vi "Main.vi"(11 "Module Admin":refnum<class "Delacor_lib_QMH_Module Admin.lvclass">) -> ()   [LabVIEW 2019, in "Aquisition.lvlib"]
doc: "This template is based off of the Queued Message Handler design pattern and the Queued Message Handler project template that ships with LabVIEW.\n\nThe main difference is that the queue is private to this module and communication between modules is performed via Broadcast and Request events.\n\nRequest events are wrapped in public API methods and are handled in the Event Handling Loop (EHL) of this VI. Any module can register for Broadcast events sent by this module. The EHL generates messages based on user interface actions.\n\nThe Message Handling Loop (MHL) processes messages generated by the EHL, or by other messages. The messages are string values, so new messages can be added easily to the Message Cases case structure in the MHL. Each message cluster can also provide an optional value for Message Data, which is a variant that can be converted to whatever message-specific data is required.\n_____\nBased on Delacor QMH Project Template 5.0.0.82."
uses:
  Aquisition.lvlib
  <vilib>/Delacor/Delacor QMH/Libraries/Module Admin_class/Delacor_lib_QMH_Module Admin.lvclass
  Module Data--cluster.ctl
  <vilib>/Delacor/Delacor QMH/Libraries/Message Queue_class/Delacor_lib_QMH_Message Queue.lvclass/Delacor_lib_QMH_Message Queue.ctl
  Stop Argument--cluster.ctl
  <vilib>/Delacor/Delacor QMH/Libraries/Module Admin_class/Delacor_lib_QMH_Module Admin.lvclass/Delacor_lib_QMH_Module Admin.ctl
  <vilib>/Utility/miscctls.llb/LVPointTypeDef.ctl
  <vilib>/Delacor/Delacor QMH/Libraries/Message Queue_class/Delacor_lib_QMH_Enqueue Message (Single).vi
  <vilib>/Delacor/Delacor QMH/Libraries/Module Admin_class/Delacor_lib_QMH_Get External Launch.vi
  <vilib>/Utility/error.llb/Error Cluster From Error Code.vi
  <vilib>/ErrorRing/Error Ring.xnode
  <vilib>/Delacor/Delacor QMH/Libraries/Message Queue_class/Delacor_lib_QMH_Message Queue.lvclass
panel:
  in  "Simulate MHL Error":bool
  in  "Simulate EHL Error":bool
  out "error out":errorcluster
  out "Status":string
  # "Other QMH Modules communicate with this Module via its Public API (wrappers for its Request Events).\n\nThis Module communicates with other Modules via its Broadcast Events.\nAny module that wants to get these messages, just registers for this module's Broadcast events."
  # "This template is for the Delacor Modified Queued Message Handler design pattern.\n\nSee the block diagram for more information on how to use this template."
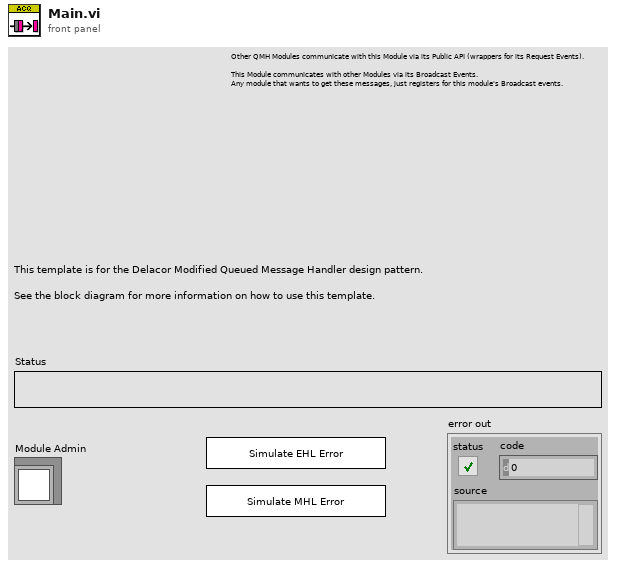
[diagram p1: front panel]
types:
  T1 = typedef "Aquisition.lvlib/Request Events--cluster.ctl" = cluster{"Stop Module":refnum<user-event>, "Show Panel":refnum<user-event>, "Hide Panel":refnum<user-event>, "Get Module Execution Status":refnum<user-event>, "Show Diagram":refnum<user-event>}
  T2 = typedef "Aquisition.lvlib/Module Data--cluster.ctl" = cluster{"Status":string}
  T3 = enum32{"invalid lock state", "Not Locked", "Locked (No Password)", "Password-protected"}
  T4 = typedef "Aquisition.lvlib/Stop Argument--cluster.ctl" = cluster{"Origin":string, "Exit via Stop Module Req?":bool, "Wait for Module to stop?":bool}
  T5 = typedef "LVPointTypeDef.ctl" = cluster{"Horizontal":i16, "Vertical":i16}
  T6 = enum32{"Invalid", "Standard", "Closed", "Hidden", "Minimized", "Maximized"}
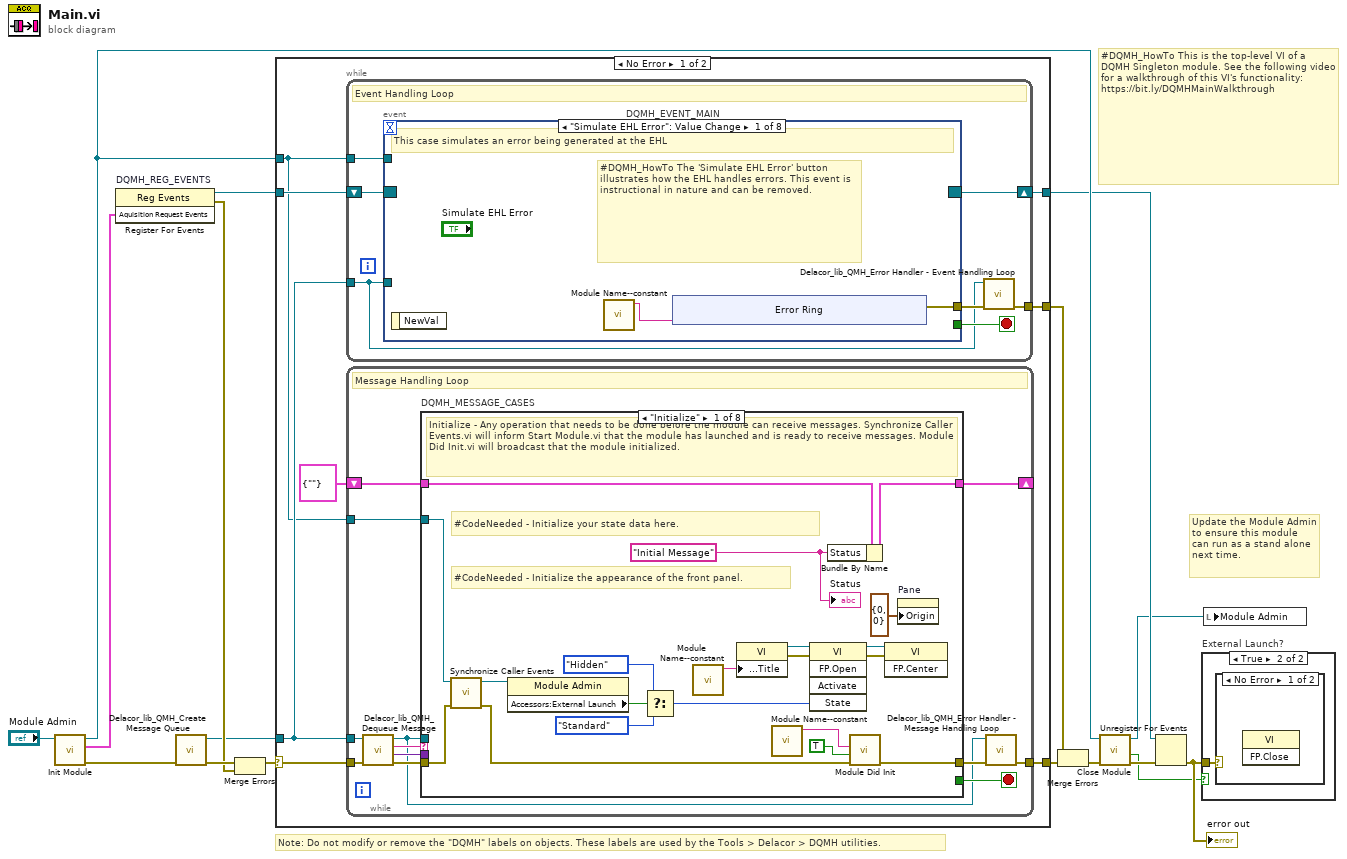
[diagram p0: block diagram]
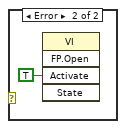
[diagram p3: hidden frame]
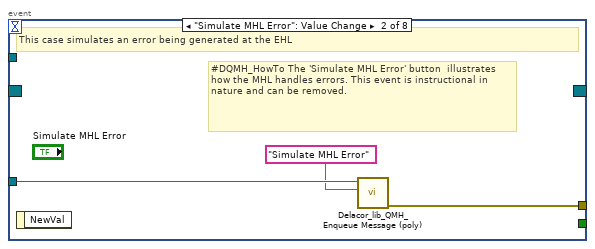
[diagram p4: hidden frame]
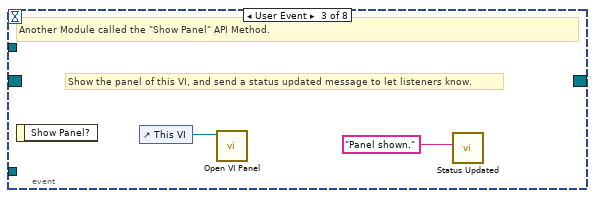
[diagram p5: hidden frame]
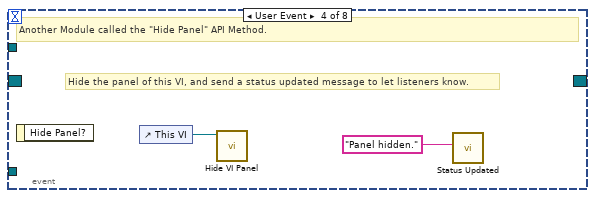
[diagram p6: hidden frame]
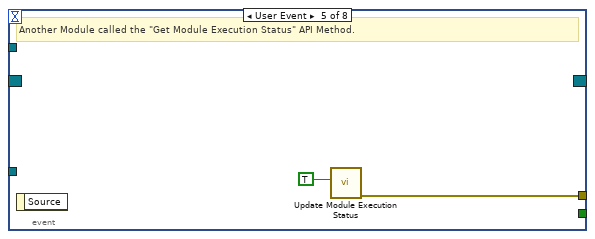
[diagram p7: hidden frame]
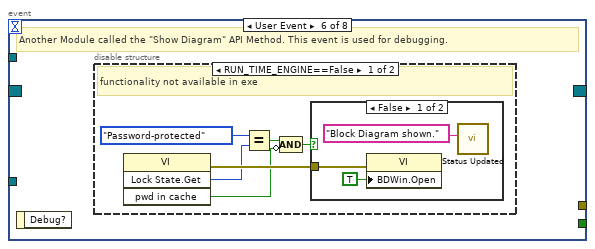
[diagram p8: hidden frame]
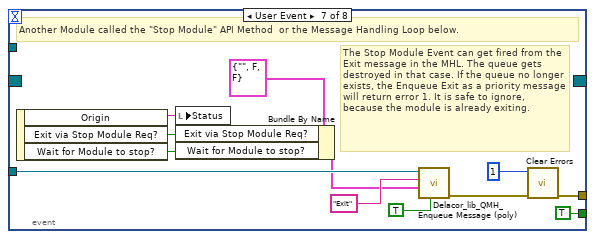
[diagram p11: hidden frame]
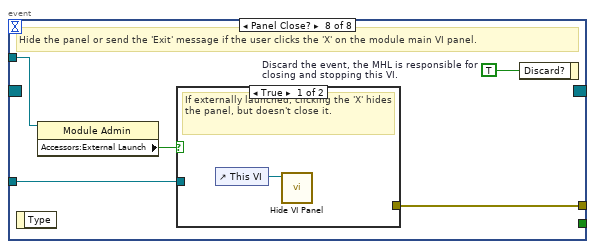
[diagram p12: hidden frame]
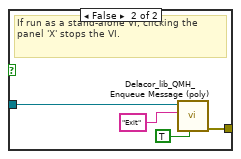
[diagram p13: hidden frame]
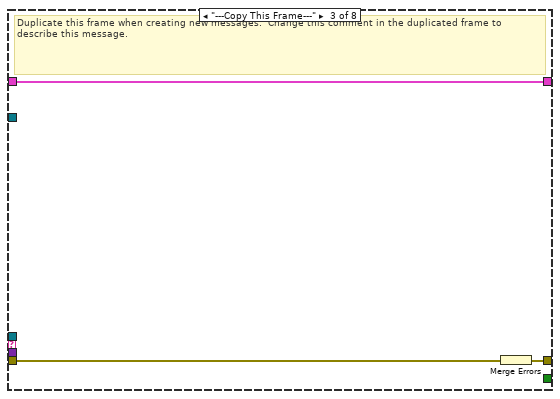
[diagram p15: hidden frame]
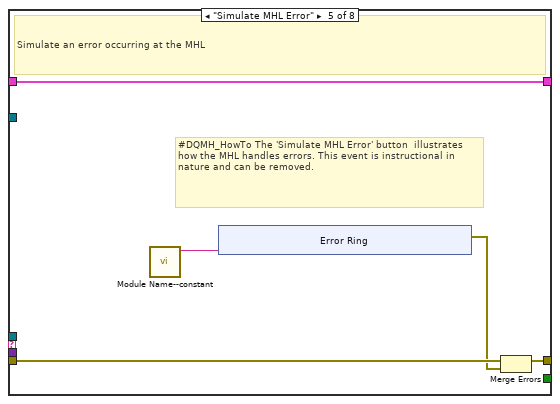
[diagram p17: hidden frame]
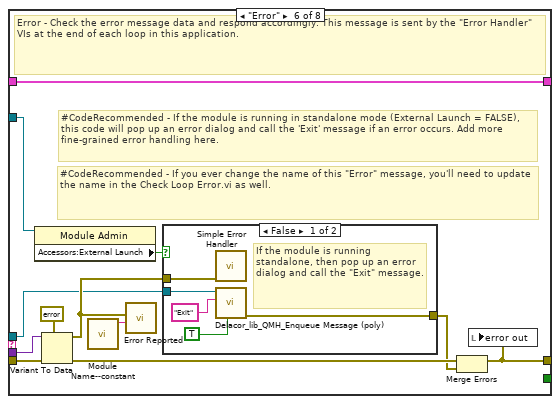
[diagram p18: hidden frame]
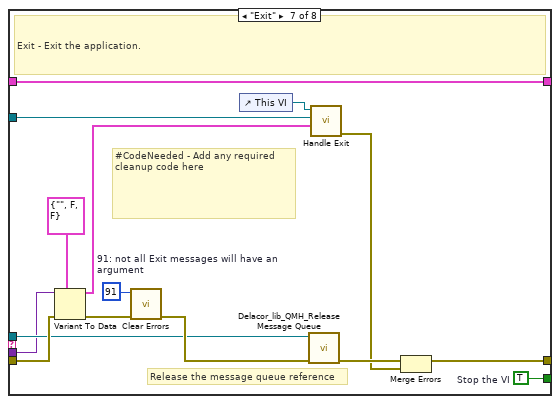
[diagram p20: hidden frame]
diagram:
  # "#DQMH_HowTo This is the top-level VI of a DQMH Singleton module. See the following video for a walkthrough of this VI's functionality: https://bit.ly/DQMHMainWalkthrough"
  # "Note: Do not modify or remove the \"DQMH\" labels on objects. These labels are used by the Tools > Delacor > DQMH utilities."
  # "Update the Module Admin to ensure this module can run as a stand alone next time."
  n1 = call "Init Module.vi"("Singleton Module Admin in"="Module Admin") -> ("error out"=w16:errorcluster, "Aquisition Request Events"=w5:T1, "Singleton Module Admin out"=w8:refnum<class "Delacor_lib_QMH_Module Admin.lvclass">)  [unwired: 8 in]
  n2 = register-events "DQMH_REG_EVENTS"(w5) -> (reference out=w6:refnum<event-registration>, error out=w9:errorcluster)  [unwired: 2 in]
  n3 = call <vilib>:"Delacor_lib_QMH_Create Message Queue.vi"("error in (no error)"=w16) -> ("error out"=w11:errorcluster, "Message Queue"=w4:refnum<class "Delacor_lib_QMH_Message Queue.lvclass">)  [unwired: 9 in]
  n4 = Merge Errors(w11, w9) -> (w10:errorcluster)
  n5 = case shown="No Error" w10 {
    selector: w10 -> [w23 w181]
    tunnel: [w25 w180] -> w17
    tunnel: [w22 w186] -> w7
    tunnel: w6 -> [w20 w186]
    tunnel: w4 -> [w19 w179]
    tunnel: [w24 _] -> w14
    tunnel: w8 -> [w18 w182]
    frame No Error {
      n6 = while {
        tunnel: w19 -> [w26]
        shift-right: [w29] -> w22
        shift-left: w20 -> [w30]
        tunnel: [w31] -> w24
        tunnel: w18 -> [w27]
        stop <- w28 stop-if-true
        # "Event Handling Loop"
        n7 = event "DQMH_EVENT_MAIN" shown="[0] \"Simulate EHL Error\": Value Change" {
          selector: w30 -> [_ _ _ _ _ _ _ _]
          dyn-events: [_ _ _ _ _ _ _ _] -> w29
          timeout: _ -> [_ _ _ _ _ _ _ _]
          tunnel: [_ _ _ _ _ _ TRUE ("Discard?") _] -> w28
          tunnel: w26 -> [_ w43 _ _ _ _ w67 w74]
          tunnel: [w34 w44 _ _ w50 _ w70 w76] -> w32
          tunnel: w27 -> [_ _ _ _ _ _ _ w73]
          event "Simulate EHL Error": Value Change {
            # "#DQMH_HowTo The 'Simulate EHL Error' button  illustrates how the EHL handles errors. This event is instructional in nature and can be removed."
            # "This case simulates an error being generated at the EHL"
            n8 = event-data() -> ()  [unwired: 1 in, 1 out]
            n9 = call "Module Name--constant.vi"() -> ("Module Name"=w33:string)  [unwired: 11 in]
            n10 = xnode "Error Ring"("parameter 0"=w33) -> ("error out"=w34:errorcluster)
          }
          event "Simulate MHL Error": Value Change {
            # "#DQMH_HowTo The 'Simulate MHL Error' button  illustrates how the MHL handles errors. This event is instructional in nature and can be removed."
            # "This case simulates an error being generated at the EHL"
            n11 = event-data() -> ()  [unwired: 1 in, 1 out]
            n12 = call-poly <vilib>:"Delacor_lib_QMH_Enqueue Message (poly).vi"("Message"="Simulate MHL Error", "Message Queue in"=w43) -> ("error out"=w44:errorcluster)  [unwired: 8 in, 1 out]
          }
          event User Event {
            # "Show the panel of this VI, and send a status updated message to let listeners know."
            # "Another Module called the \"Show Panel\" API Method."
            n13 = event-data() -> ()  [unwired: 1 in, 1 out]
            n14 = control-ref of="This VI"() -> (w46:refnum<vi>)
            n15 = call "Open VI Panel.vi"("VI"=w46) -> ()  [unwired: 10 in, 1 out]
            n16 = call "Status Updated.vi"("Status"="Panel shown." ("format string")) -> ()  [unwired: 10 in, 1 out]
          }
          event User Event {
            # "Hide the panel of this VI, and send a status updated message to let listeners know."
            # "Another Module called the \"Hide Panel\" API Method."
            n17 = event-data() -> ()  [unwired: 1 in, 1 out]
            n18 = control-ref of="This VI"() -> (w48:refnum<vi>)
            n19 = call "Hide VI Panel.vi"("VI"=w48) -> ()  [unwired: 10 in, 1 out]
            n20 = call "Status Updated.vi"("Status"="Panel hidden." ("format string")) -> ()  [unwired: 10 in, 1 out]
          }
          event User Event {
            # "Another Module called the \"Get Module Execution Status\" API Method."
            n21 = event-data() -> ()  [unwired: 1 in, 1 out]
            n22 = call "Update Module Execution Status.vi"("Running?"=TRUE) -> ("error out"=w50:errorcluster)  [unwired: 10 in]
          }
          event User Event {
            # "Another Module called the \"Show Diagram\" API Method. This event is used for debugging."
            n23 = event-data() -> ()  [unwired: 1 in, 1 out]
            n24 = disable-structure shown="RUN_TIME_ENGINE==False" {
              frame condition #0 (active) {
                # "functionality not available in exe"
                n25 = invoke class="VI" method="Lock State.Get"() -> (error out=w56:errorcluster, "Get Lock State"=w55:T3, "pwd in cache"=w52:bool)  [unwired: 4 in, 1 out]
                n26 = Equal?(x=T3."Password-protected", y=w55) -> (x = y?=w53:bool)
                n27 = Compound Arithmetic op=AND(w53, invert w52) -> (w51:bool)
                n28 = case shown="False" w51 {
                  tunnel: w56 -> [w59 _]
                  frame False {
                    n29 = property class="VI"(error in=w59, "BDWin.Open"=TRUE ("Block Diagram Window:Open")) -> ()  [unwired: 1 in, 2 out]
                    n30 = call "Status Updated.vi"("Status"="Block Diagram shown." ("format string")) -> ()  [unwired: 10 in, 1 out]
                  }
                  frame True {
                    # "Password-protected VI, and the password is not in the cache. Do not show the diagram."
                  }
                }
              }
              frame condition #1 {
              }
            }
          }
          event User Event {
            # "The Stop Module Event can get fired from the Exit message in the MHL. The queue gets destroyed in that case. If the queue no longer exists, the Enqueue Exit as a priority message will return error 1. It is safe to ignore, because the module is already exiting."
            # "Another Module called the \"Stop Module\" API Method  or the Message Handling Loop below."
            n31 = event-data() -> ("Origin"=w66:string, "Exit via Stop Module Req?"=w62:bool, "Wait for Module to stop?"=w61:bool)  [unwired: 1 in]
            n32 = local write "Status"(w66) -> ()
            n33 = Bundle By Name(cluster=T4 {"Origin"="", "Exit via Stop Module Req?"=FALSE, "Wait for Module to stop?"=FALSE} ("Stop Argument"), "Exit via Stop Module Req?"=w62, "Wait for Module to stop?"=w61) -> (w60:T4)
            n34 = call-poly <vilib>:"Delacor_lib_QMH_Enqueue Message (poly).vi"("Priority Message? (F)"=TRUE, "Message Data"=w60, "Message"="Exit", "Message Queue in"=w67) -> ("error out"=w71:errorcluster)  [unwired: 6 in, 1 out]
            n35 = call <vilib>:"Clear Errors.vi"("error in (no error)"=w71, "specific error code to clear (0: all)"=1) -> ("error out"=w70:errorcluster)  [unwired: 4 in, 1 out]
          }
          event Panel Close? {
            w75 = TRUE  # Discard the event, the MHL is responsible for closing and stopping this VI.
            # "Hide the panel or send the 'Exit' message if the user clicks the 'X' on the module main VI panel."
            n36 = event-data() -> ()  [unwired: 1 in, 1 out]
            n37 = property class="Module Admin"(reference=w73) -> ("Accessors:External Launch"=w72:bool)  [unwired: 1 in, 2 out]
            n38 = case shown="True" w72 {
              tunnel: w74 -> [_ w80]
              tunnel: [_ w81] -> w76
              frame True {
                # "If externally launched, clicking the 'X' hides the panel, but doesn't close it."
                n39 = control-ref of="This VI"() -> (w77:refnum<vi>)
                n40 = call "Hide VI Panel.vi"("VI"=w77) -> ()  [unwired: 10 in, 1 out]
              }
              frame False {
                # "If run as a stand-alone VI, clicking the panel 'X' stops the VI."
                n41 = call-poly <vilib>:"Delacor_lib_QMH_Enqueue Message (poly).vi"("Priority Message? (F)"=TRUE, "Message"="Exit", "Message Queue in"=w80) -> ("error out"=w81:errorcluster)  [unwired: 7 in, 1 out]
              }
            }
            n42 = event-data("Discard?"=w75) -> ()  [unwired: 1 in, 1 out]
          }
        }
        n43 = call-dynamic "Delacor_lib_QMH_Error Handler - Event Handling Loop.vi"("error in (no error)"=w32, "Message Queue in"=w26) -> ("dup error in"=w31:errorcluster)  [unwired: 8 in, 1 out]
      }
      n44 = while {
        tunnel: w19 -> [w84]
        shift-right: [w88] -> _
        shift-left: T2 {"Status"=""} ("Data Cluster") -> [w89]
        tunnel: w23 -> [w92]
        tunnel: [w90] -> w25
        tunnel: w18 -> [w82]
        stop <- w87 stop-if-true
        # "Message Handling Loop"
        n45 = call-dynamic "Delacor_lib_QMH_Dequeue Message.vi"("error in (no error)"=w92, "Message Queue in"=w84) -> ("error out"=w91:errorcluster, "Message Data"=w85:variant, "Message"=w86:string, "Message Queue out"=w83:refnum<class "Delacor_lib_QMH_Message Queue.lvclass">)  [unwired: 6 in]
        n46 = case "DQMH_MESSAGE_CASES" shown="\"Initialize\"" w86 {
          selector: w86 -> [_ _ _ _ _ _ _ w166]
          tunnel: w83 -> [_ _ _ _ _ w136 w158 _]
          tunnel: w91 -> [w111 w115 w118 w120 w125 w143 w164 w168]
          tunnel: [w109 w115 w117 w120 w124 w139 w161 w169] -> w93
          tunnel: w89 -> [w100 w114 w116 w119 w122 w138 w157 w167]
          tunnel: [w99 w114 w116 w119 w122 w138 w157 w167] -> w88
          tunnel: [_ _ _ _ _ _ w156 _] -> w87
          tunnel: w85 -> [_ _ _ _ _ w137 w155 _]
          tunnel: w82 -> [w101 _ _ _ _ w135 w150 _]
          frame "Initialize" {
            w94 = "Initial Message" ("Initial Message")
            # "#CodeNeeded - Initialize the appearance of the front panel."
            # "#CodeNeeded - Initialize your state data here."
            # "Initialize - Any operation that needs to be done before the module can receive messages. Synchronize Caller Events.vi will inform Start Module.vi that the module has launched and is ready to receive messages. Module Did Init.vi will broadcast that the module initialized."
            n47 = call "Synchronize Caller Events.vi"("error in (no error)"=w111, "Singleton Module Admin in"=w101) -> ("error out"=w110:errorcluster, "Singleton Module Admin out"=w96:refnum<class "Delacor_lib_QMH_Module Admin.lvclass">)  [unwired: 8 in]
            n48 = property class="Module Admin"(reference=w96) -> ("Accessors:External Launch"=w105:bool)  [unwired: 1 in, 2 out]
            n49 = Select(t=T6."Hidden" ("State"), s=w105, f=T6."Standard" ("State")) -> (s? t:f=w102:T6)
            n50 = call "Module Name--constant.vi"() -> ("Module Name"=w108:string)  [unwired: 11 in]
            n51 = property class="VI"("Front Panel.Title"=w108) -> (reference out=w107:refnum<vi>, error out=w113:errorcluster)  [unwired: 2 in]
            n52 = call "Module Name--constant.vi"() -> ("Module Name"=w97:string)  [unwired: 11 in]
            n53 = invoke class="VI" method="FP.Open"(reference=w107, error in=w113, "State"=w102) -> (reference out=w106:refnum<vi>, error out=w112:errorcluster)  [unwired: 2 in, 3 out]
            n54 = Bundle By Name(cluster=w100, "Status"=w94) -> (w99:T2)
            n55 = call "Module Did Init.vi"("error in (no error)"=w110, "Initialized?"=TRUE, "Origin"=w97) -> ("error out"=w109:errorcluster)  [unwired: 8 in]
            n56 = invoke class="VI" method="FP.Center"(reference=w106, error in=w112) -> ()  [unwired: 1 in, 3 out]
            n57 = property on="Pane" class="Pane"("Origin"=T5 {"Horizontal"=0, "Vertical"=0}) -> ()  [unwired: 2 in, 2 out]
            "Status" <- w94
          }
          frame "--- Module Specific ---" {
            # "Separator -- The following cases handle messages specific to this Module."
          }
          frame "---Copy This Frame---" {
            # "Duplicate this frame when creating new messages.  Change this comment in the duplicated frame to describe this message."
            n58 = Merge Errors(w118) -> (w117:errorcluster)
          }
          frame "--- Exit and Error Handling---" {
            # "Separator - The following cases handle errors and exit messages."
          }
          frame "Simulate MHL Error" {
            # "#DQMH_HowTo The 'Simulate MHL Error' button  illustrates how the MHL handles errors. This event is instructional in nature and can be removed."
            # "Simulate an error occurring at the MHL"
            n59 = call "Module Name--constant.vi"() -> ("Module Name"=w121:string)  [unwired: 11 in]
            n60 = xnode "Error Ring"("parameter 0"=w121) -> ("error out"=w123:errorcluster)
            n61 = Merge Errors(w125, w123) -> (w124:errorcluster)
          }
          frame "Error" {
            # "#CodeRecommended - If you ever change the name of this \"Error\" message, you'll need to update the name in the Check Loop Error.vi as well."
            # "#CodeRecommended - If the module is running in standalone mode (External Launch = FALSE), this code will pop up an error dialog and call the 'Exit' message if an error occurs. Add more fine-grained error handling here."
            # "Error - Check the error message data and respond accordingly. This message is sent by the \"Error Handler\" VIs at the end of each loop in this application."
            n62 = property class="Module Admin"(reference=w135) -> ("Accessors:External Launch"=w134:bool)  [unwired: 1 in, 2 out]
            n63 = Variant To Data(error in=w143, type=errorcluster {"status"=FALSE, "code"=0, "source"=""} ("error constant"), Variant=w137) -> (data=w144:errorcluster, error out=w141:errorcluster)
            n64 = call "Module Name--constant.vi"() -> ("Module Name"=w133:string)  [unwired: 11 in]
            n65 = call "Error Reported.vi"("Additional Information"=w133, "Error"=w144) -> ()  [unwired: 9 in, 1 out]
            n66 = case shown="False" w134 {
              tunnel: [w149 _] -> w140
              tunnel: w136 -> [w147 _]
              tunnel: w144 -> [w148 _]
              frame False {
                # "If the module is running standalone, then pop up an error dialog and call the \"Exit\" message."
                n67 = call <vilib>:"Simple Error Handler.vi"("error in (no error)"=w148) -> ()  [unwired: 4 in, 5 out]
                n68 = call-poly <vilib>:"Delacor_lib_QMH_Enqueue Message (poly).vi"("Priority Message? (F)"=TRUE, "Message"="Exit", "Message Queue in"=w147) -> ("error out"=w149:errorcluster)  [unwired: 7 in, 1 out]
              }
              frame True {
                # "If the module was launched externally, calling the Error Reported broadcast VI is the only action performed by the \"Error\" message. The module's caller can then process the error appropriately."
              }
            }
            n69 = Merge Errors(w141, w140) -> (w139:errorcluster)
            n70 = local write "error out"(w139) -> ()
          }
          frame "Exit" {
            w154 = 91  # 91: not all Exit messages will have an argument
            w156 = TRUE  # Stop the VI
            # "Release the message queue reference"
            # "#CodeNeeded - Add any required cleanup code here"
            # "Exit - Exit the application."
            n71 = Variant To Data(error in=w164, type=T4 {"Origin"="", "Exit via Stop Module Req?"=FALSE, "Wait for Module to stop?"=FALSE} ("Stop Argument"), Variant=w155) -> (data=w152:T4, error out=w160:errorcluster)
            n72 = call <vilib>:"Clear Errors.vi"("error in (no error)"=w160, "specific error code to clear (0: all)"=w154) -> ("error out"=w163:errorcluster)  [unwired: 4 in, 1 out]
            n73 = control-ref of="This VI"() -> (w151:refnum<vi>)
            n74 = call-dynamic "Delacor_lib_QMH_Release Message Queue.vi"("error in (no error)"=w163, "Message Queue"=w158) -> ("error out"=w162:errorcluster)  [unwired: 9 in]
            n75 = call "Handle Exit.vi"("Stop Argument"=w152, "Admin in"=w150, "VI reference"=w151) -> ("error out"=w159:errorcluster)  [unwired: 7 in, 1 out]
            n76 = Merge Errors(w162, w159) -> (w161:errorcluster)
          }
          frame Default {
            # "'Default' case only runs if there is a message that isn't defined in any of the other cases.  Output a programming error."
            n77 = call "Module Name--constant.vi"() -> ("Module Name"=w165:string)  [unwired: 11 in]
            n78 = xnode "Error Ring"("parameter 0"=w166, "parameter 1"=w165) -> ("error out"=w170:errorcluster)
            n79 = Merge Errors(w168, w170) -> (w169:errorcluster)
          }
        }
        n80 = call-dynamic "Delacor_lib_QMH_Error Handler - Message Handling Loop.vi"("error in (no error)"=w93, "Message Queue in"=w83) -> ("dup error in"=w90:errorcluster)  [unwired: 8 in, 1 out]
      }
    }
    frame Error {
      # "Synchronize Caller Events.vi will inform Start Module.vi that the module has launched and will let the code calling Start Module.vi register for broadcasts and would permit the caller receive the broadcast that an error occurred at launch time."
      n81 = call-dynamic "Delacor_lib_QMH_Release Message Queue.vi"("error in (no error)"=w181, "Message Queue"=w179) -> ("error out"=w180:errorcluster)  [unwired: 9 in]
      n82 = call "Synchronize Caller Events.vi"("Singleton Module Admin in"=w182) -> ("error out"=w187:errorcluster)  [unwired: 9 in, 1 out]
      n83 = call "Module Name--constant.vi"() -> ("Module Name"=w185:string)  [unwired: 11 in]
      n84 = Format Into String(format string="An error occurred during initialization. %s is no longer running.", w185) -> (resulting string=w183:string)  [unwired: 2 in, 1 out]
      n85 = Merge Errors(w180, w187) -> (w188:errorcluster)
      n86 = call "Error Reported.vi"("Additional Information"=w183, "Error"=w188) -> ()  [unwired: 9 in, 1 out]
    }
  }
  n87 = Merge Errors(w14, w17) -> (w13:errorcluster)
  n88 = call "Close Module.vi"("error in (no error)"=w13, "Module Admin in"=w8) -> ("error out"=w15:errorcluster, "External Launch"=w1:bool, "Module Admin out"=w2:refnum<class "Delacor_lib_QMH_Module Admin.lvclass">)  [unwired: 7 in]
  n89 = Unregister For Events(event registration refnum=w7, error in=w15) -> (error out=w12:errorcluster)
  "error out" <- w12
  n90 = case "External Launch?" shown="True" w1 {
    tunnel: w12 -> [_ w189]
    frame False {
    }
    frame True {
      n91 = case shown="No Error" w189 {
        frame No Error {
          n92 = invoke class="VI" method="FP.Close"() -> ()  [unwired: 3 in, 3 out]
        }
        frame Error {
          n93 = invoke class="VI" method="FP.Open"("Activate"=TRUE ("Activate?")) -> ()  [unwired: 4 in, 5 out]
        }
      }
    }
  }
  n94 = local write "Module Admin"(w2) -> ()
